vi "Set Popout Event.vi"(8 "error in (no error)":errorcluster, 10 "Popout Nav Event":refnum<user-event>, 11 "NavPanel in":refnum<class "NavPanel.lvclass">) -> (0 "error out":errorcluster, 3 "NavPanel out":refnum<class "NavPanel.lvclass">)   [LabVIEW 2020, in "PicoG-App.lvlib" / "NavPanel.lvclass"]
uses:
  NavPanel.lvclass
  <vilib>/IlluminatedG/IG OOPanel/OOPanel/Panel/Panel.lvclass
  Popout Nav Panel Event.ctl
  PicoG-App.lvlib
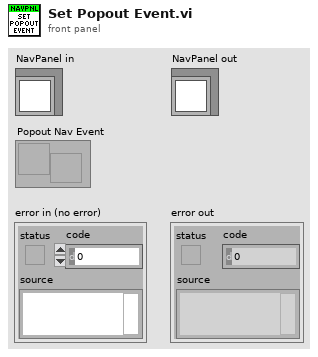
[diagram p1: front panel]
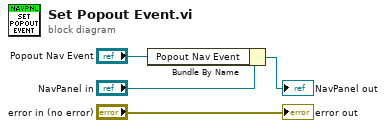
[diagram p0: block diagram]
diagram:
  n1 = Bundle By Name(cluster="NavPanel in", "Popout Nav Event"="Popout Nav Event") -> (→"NavPanel out":refnum<class "NavPanel.lvclass">)
  "error out" <- "error in (no error)"
